vi "Configure Frequency.vi"(8 "error in (no error)":errorcluster, 10 "Frequency [Hz]":dbl, 11 "PSG-MXG in":refnum<class "PSG-MXG.lvclass">) -> (0 "error out":errorcluster, 3 "PSG-MXG out":refnum<class "PSG-MXG.lvclass">)   [LabVIEW 2020, in "PSG-MXG.lvclass"]
uses:
  PSG-MXG.lvclass
  C:/Sandbox/RF Bench/Source Code/WiSpry Test Framework/Instruments/Instrument.lvclass
  C:/Sandbox/RF Bench/Source Code/WiSpry Test Framework/Instruments/Signal Generator/Signal Generator.lvclass
  Instrument.lvclass/Instrument.ctl
  Signal Generator.lvclass/Signal Generator.ctl
  Instrument.lvclass
  <instrlib>/Agilent PSG MXG Series/Agilent PSG MXG Series.lvlib
  Signal Generator.lvclass
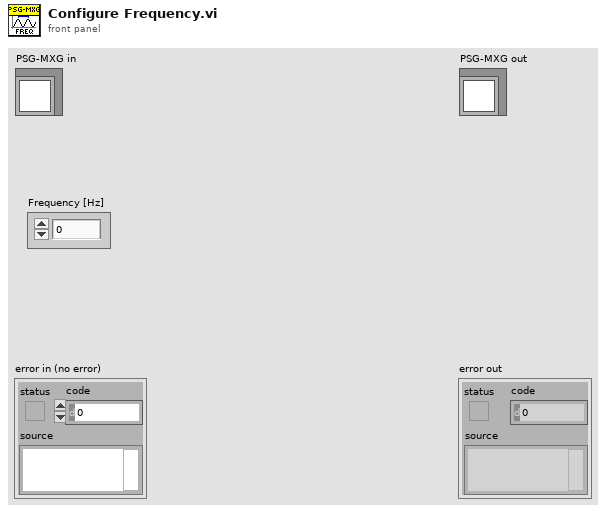
[diagram p1: front panel]
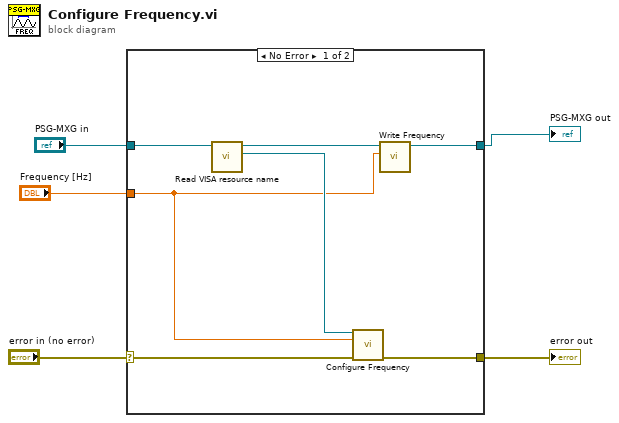
[diagram p0: block diagram]
diagram:
  n1 = case shown="No Error" "error in (no error)" {
    selector: "error in (no error)" -> [w10 w14]
    tunnel: "PSG-MXG in" -> [w12 w13]
    tunnel: [w9 w14] -> w4
    tunnel: [w7 w13] -> w3
    tunnel: "Frequency [Hz]" -> [w6 _]
    frame No Error {
      n2 = call "Read VISA resource name.vi"("Instrument in"=w12) -> ("VISA resource name"=w11:refnum<visa-resource-name>, "Instrument out"=w8:refnum<class "PSG-MXG.lvclass">)  [unwired: 9 in]
      n3 = call <instrlib>:"Configure Frequency.vi"("VISA resource name"=w11, "Frequency (100 kHz)"=w6, "error in (no error)"=w10) -> ("error out"=w9:errorcluster)  [unwired: 11 in, 1 out]
      n4 = call "Write Frequency.vi"("Frequency"=w6, "Signal Generator in"=w8) -> ("Signal Generator out"=w7:refnum<class "PSG-MXG.lvclass">)  [unwired: 9 in]
    }
    frame Error {
    }
  }
  "error out" <- w4
  "PSG-MXG out" <- w3
